vi "UHR-Fleezers Control (host) - 11.0.vi"() -> ()   [LabVIEW 2011] (continued)
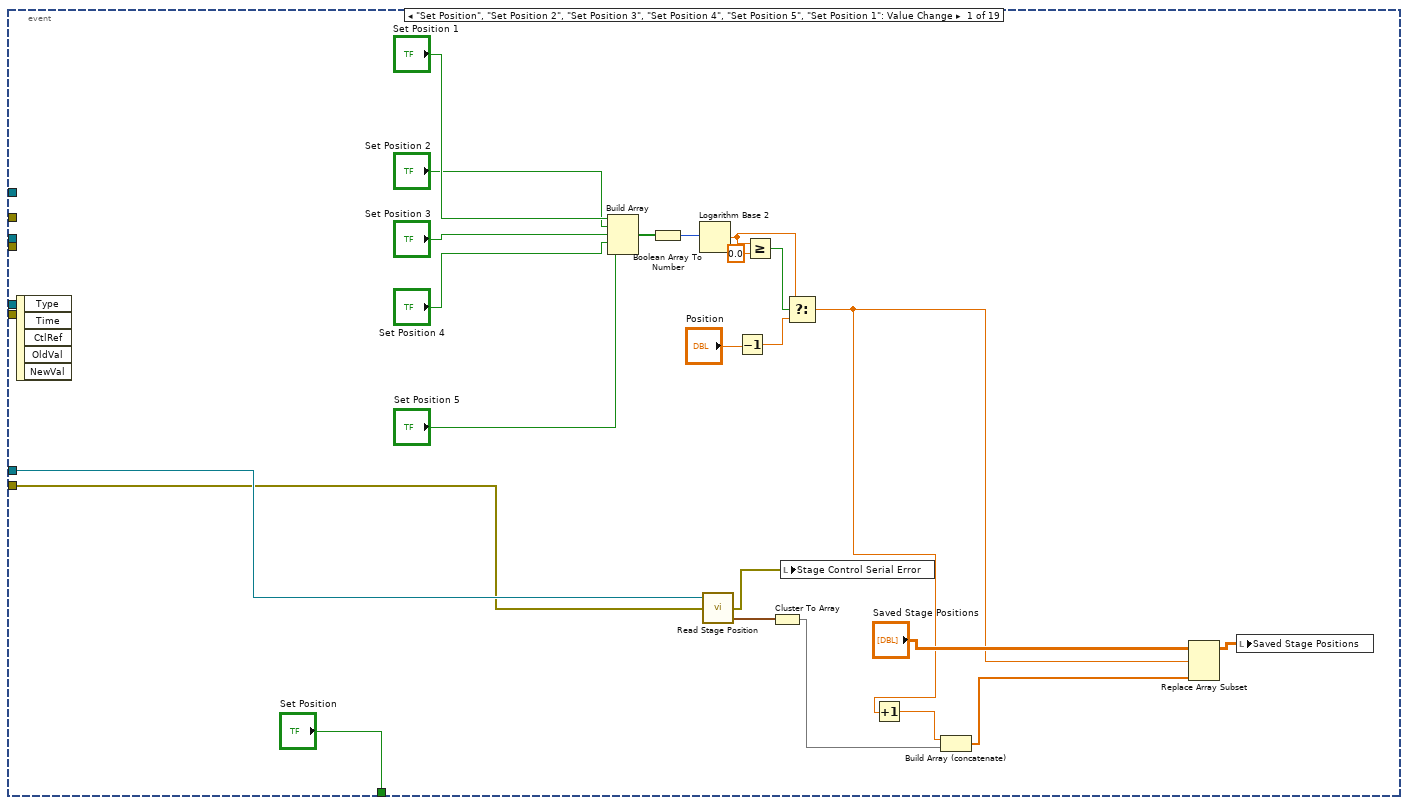
[diagram p2: hidden frame]
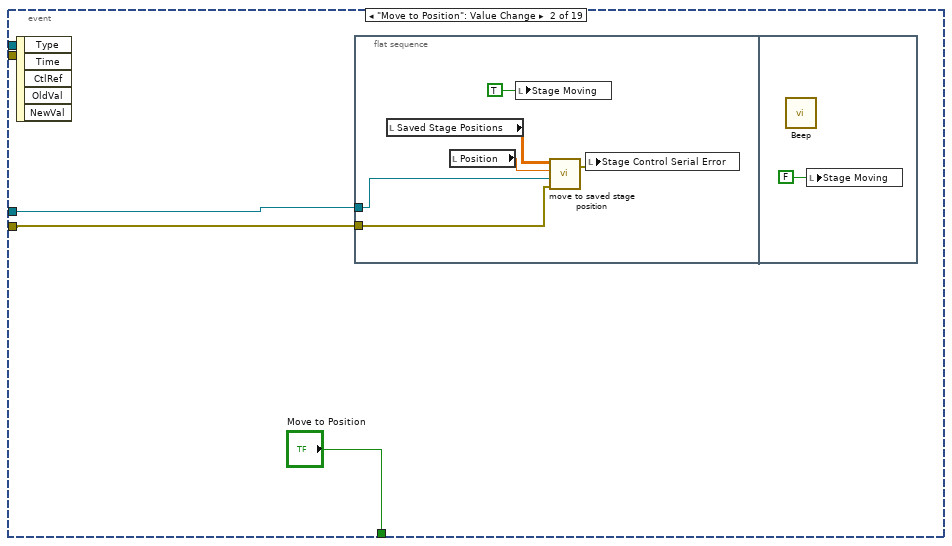
[diagram p3: hidden frame]
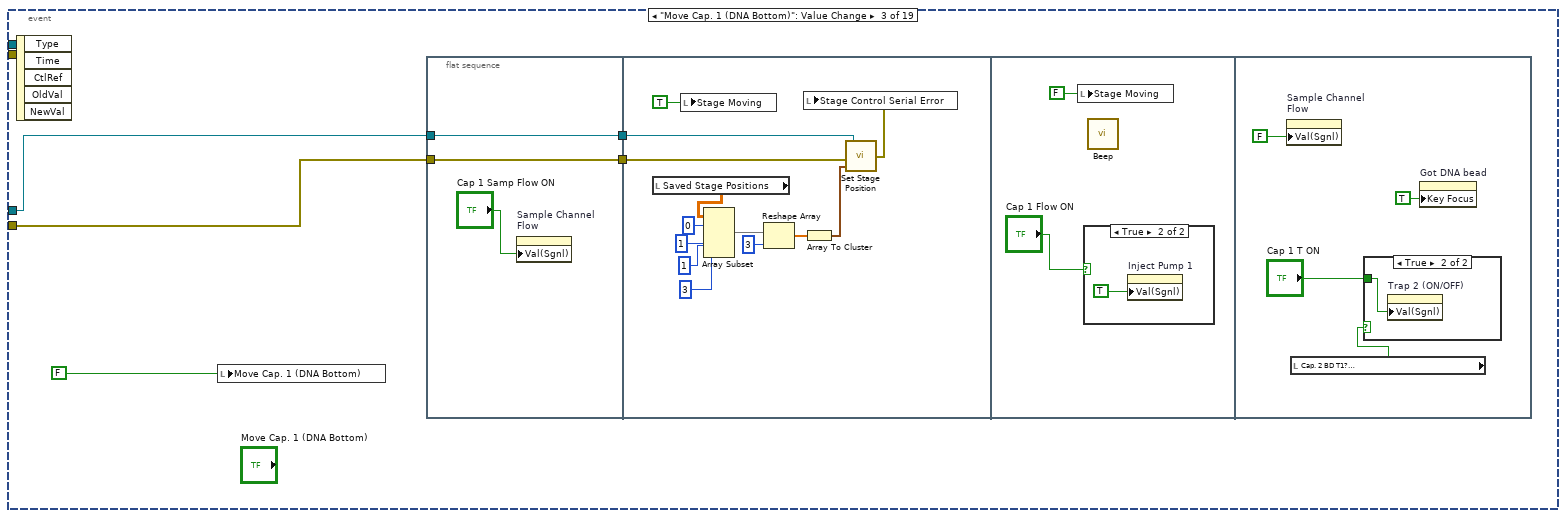
[diagram p4: hidden frame]
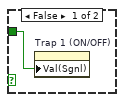
[diagram p6: hidden frame]
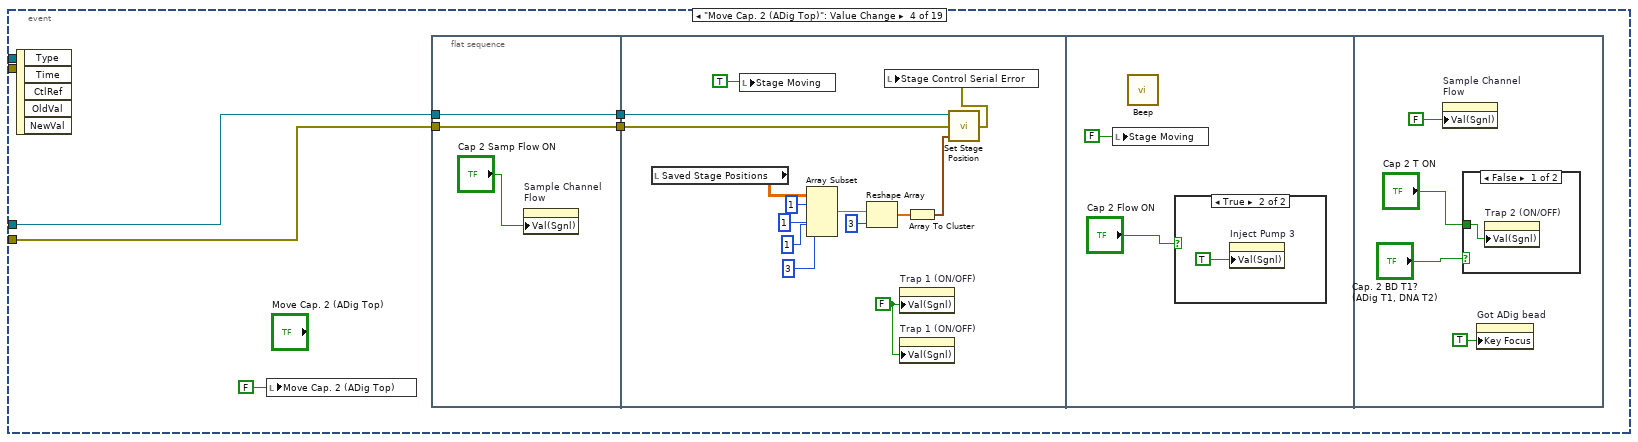
[diagram p7: hidden frame]
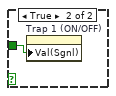
[diagram p9: hidden frame]
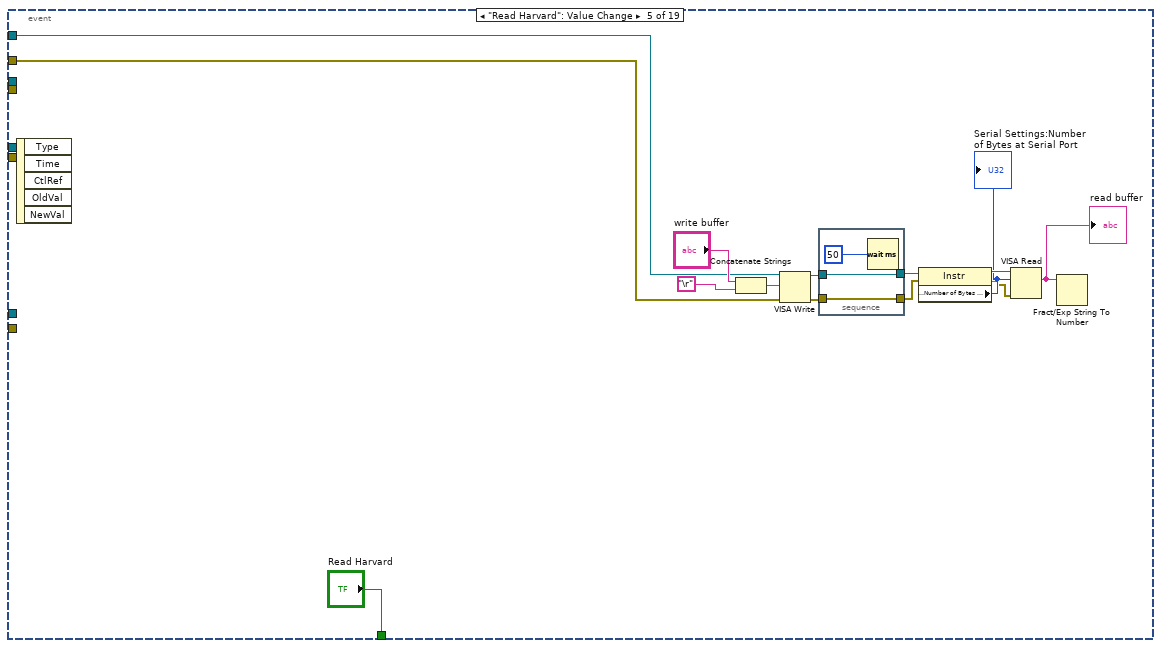
[diagram p10: hidden frame]
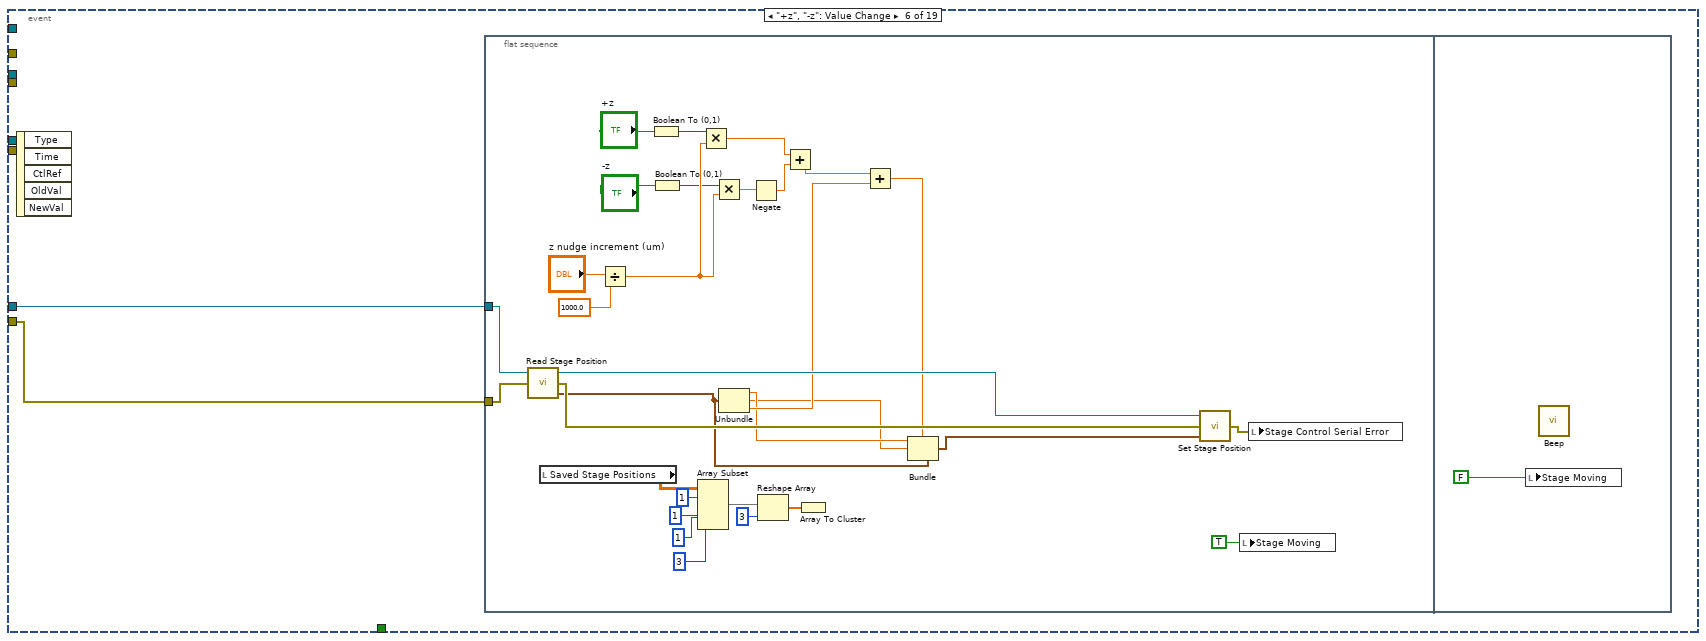
[diagram p11: hidden frame]
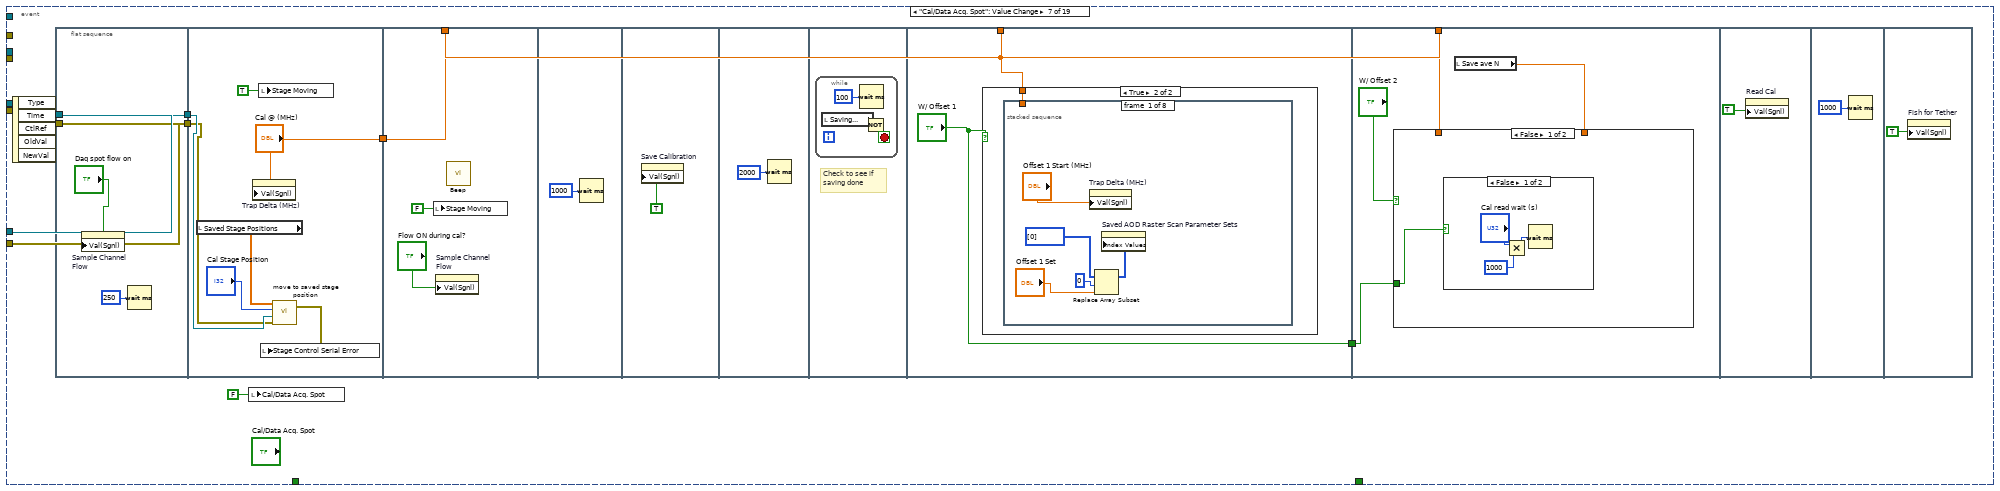
[diagram p12: hidden frame]
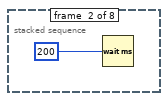
[diagram p14: hidden frame]
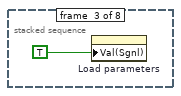
[diagram p15: hidden frame]
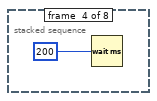
[diagram p16: hidden frame]
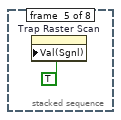
[diagram p17: hidden frame]
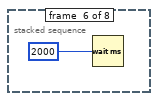
[diagram p18: hidden frame]
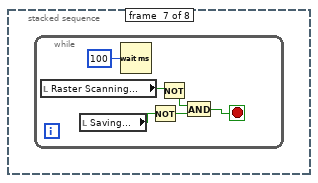
[diagram p19: hidden frame]
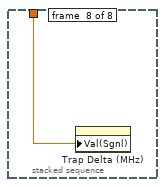
[diagram p20: hidden frame]
                n2907 = Build Array(w4669, w4664, w4662, w4660, w4659, w4650, w4649) -> (w4666:dbl[])
                n2908 = Build Array(w4651, w4655, w4675, w4674, w4673, 3.0 ("t")) -> (w4668:dbl[])
                n2909 = Round Toward +Infinity(x=w4657) -> (ceil(x): smallest int >= x=w4658:dbl)
                n2910 = Build Array (concatenate)(w4668, w4667, w4652, w4666) -> (w4665:dbl[])
                n2911 = To Unsigned Long Integer(number=w4658) -> (unsigned 32bit integer=w4656:u32)
              }
            }
            n2912 = local read "Index"() -> (w4515:dbl)
            n2913 = call "Create new save file.vi"("Insert"="", "Ext"=".dat", "Index In"=w4515) -> ("Path Out"=w4474:path, "Index Out"=w4487:dbl)
            n2914 = local write "Save file name"(w4474) -> ()
            n2915 = local write "Index"(w4487) -> ()
            n2916 = local write "Save index"(w4487) -> ()
            n2917 = Array Size(array=w4498) -> (size(s)=w4499:i32)
            n2918 = Open/Create/Replace File(file path (use dialog)=w4474, operation (0:open)=T25."create", access (0:read/write)=enum16{"read/write", "read-only", "write-only"}."write-only") -> (refnum out=w4512:refnum<file>)  [unwired: 1 in, 4 out]
            n2919 = local write "Saving..."(TRUE ("Saving...")) -> ()
            n2920 = To Double Precision Float(number=w4499) -> (double precision float=w4497:dbl)
            n2921 = String Length(string="Comment (data description)") -> (length=w4495:i32)
            n2922 = To Double Precision Float(number=w4495) -> (double precision float=w4494:dbl)
            n2923 = Deny Access(7:w4512) -> (3:w4511:refnum<file>)  [unwired: 1 in, 2 out]
            n2924 = Build Array (concatenate)(w4497, w4498, w4494) -> (w4496:dbl[])
            n2925 = case "If fluorescence data to be saved" shown="True" w4485 {
              tunnel: w4474 -> [_ w4564]
              tunnel: [refnum<k0> refnum w4544] -> w4486
              frame False {
              }
              frame True {
                w4543 = 0.0
                n2926 = local read "APD Integration Time (s)"() -> (w4549:dbl)
                n2927 = local read "N APD Samp/step"() -> (w4542:dbl)
                n2928 = Path To String(path=w4564) -> (string=w4563:string)
                n2929 = String Length(string=w4563) -> (length=w4562:i32)
                n2930 = Subtract(x=w4562, y=4) -> (x-y=w4560:i32)
                n2931 = String Subset(string=w4563, length (rest)=w4560) -> (substring=w4559:string)  [unwired: 1 out]
                n2932 = Build Array(w4549, w4542, w4543, w4543, w4543, w4543, w4543, w4543) -> (w4546:dbl[])
                n2933 = Concatenate Strings(w4559, "_fl.dat" ("string")) -> (w4557:string)
                n2934 = Array Size(array=w4546) -> (size(s)=w4548:i32)
                n2935 = String To Path(string=w4557) -> (path=w4553:path)
                n2936 = Open/Create/Replace File(file path (use dialog)=w4553, operation (0:open)=T25."create", access (0:read/write)=enum16{"read/write", "read-only", "write-only"}."write-only") -> (refnum out=w4554:refnum<file>)  [unwired: 1 in, 4 out]
                n2937 = Deny Access(7:w4554) -> (3:w4550:refnum<file>)  [unwired: 1 in, 2 out]
                n2938 = To Double Precision Float(number=w4548) -> (double precision float=w4547:dbl)
                n2939 = Build Array (concatenate)(w4547, w4546) -> (w4545:dbl[])
                n2940 = Write to Binary File(file (use dialog)=w4550, data=w4545, 5:FALSE ("prepend array or string size? (T)"), 9:T24."big-endian, network order" ("byte order (0:big-endian, network order)")) -> (refnum out=w4544:refnum<file>)  [unwired: 1 in, 3 out]
              }
            }
            n2941 = case shown="True" w4472 {
              tunnel: w4474 -> [_ w4526]
              tunnel: [refnum<k0> refnum w4525] -> w4473
              frame False {
              }
              frame True {
                w4521 = 0.0 ("element")
                n2942 = Path To String(path=w4526) -> (string=w4540:string)
                n2943 = Build Array(w4521, w4521, w4521, w4521, w4521, w4521, w4521, w4521) -> (w4522:dbl[])
                n2944 = String Length(string=w4540) -> (length=w4539:i32)
                n2945 = Subtract(x=w4539, y=4) -> (x-y=w4537:i32)
                n2946 = Array Size(array=w4522) -> (size(s)=w4524:i32)
                n2947 = String Subset(string=w4540, length (rest)=w4537) -> (substring=w4536:string)  [unwired: 1 out]
                n2948 = To Double Precision Float(number=w4524) -> (double precision float=w4523:dbl)
                n2949 = Concatenate Strings(w4536, "_pos.dat" ("string")) -> (w4534:string)
                n2950 = Build Array (concatenate)(w4523, w4522) -> (w4520:dbl[])
                n2951 = String To Path(string=w4534) -> (path=w4530:path)
                n2952 = Open/Create/Replace File(file path (use dialog)=w4530, operation (0:open)=T25."create", access (0:read/write)=enum16{"read/write", "read-only", "write-only"}."write-only") -> (refnum out=w4531:refnum<file>)  [unwired: 1 in, 4 out]
                n2953 = Deny Access(7:w4531) -> (3:w4527:refnum<file>)  [unwired: 1 in, 2 out]
                n2954 = Write to Binary File(file (use dialog)=w4527, data=w4520, 5:FALSE ("prepend array or string size? (T)"), 9:T24."big-endian, network order" ("byte order (0:big-endian, network order)")) -> (refnum out=w4525:refnum<file>)  [unwired: 1 in, 3 out]
              }
            }
            n2955 = Write to Binary File(file (use dialog)=w4511, data=w4496, 5:w4492, 9:w4490) -> (refnum out=w4493:refnum<file>)  [unwired: 1 in, 3 out]
            n2956 = Write to Binary File(file (use dialog)=w4493, data="Comment (data description)", 5:w4492, 9:w4490) -> (refnum out=w4489:refnum<file>)  [unwired: 1 in, 3 out]
          }
        }
        n2957 = feedback-in #28(w4432) -> ()
        n2958 = feedback-in #29(w4459) -> ()
        n2959 = feedback-in #30(w4431) -> ()
        n2960 = feedback-in #31(w4442) -> ()
        n2961 = feedback-in #32(w4445) -> ()
        n2962 = feedback-in #33(w4458) -> ()
        n2963 = feedback-in #34(w4448) -> ()
      }
      frame #1 {
        n2964 = local read "Saving..."() -> (w4689:bool)
        n2965 = case shown="True" w4689 {
          tunnel: w4693 -> [_ w4703]
          tunnel: w4692 -> [_ w4717]
          tunnel: w4691 -> [_ w4713]
          tunnel: w4690 -> [_ w4712]
          tunnel: w4688 -> [_ w4711]
          tunnel: w4687 -> [_ w4706]
          tunnel: w4686 -> [_ w4705]
          tunnel: w4685 -> [_ w4704]
          tunnel: w4684 -> [_ w4702]
          tunnel: w4683 -> [_ w4700]
          tunnel: w4682 -> [_ w4699]
          tunnel: w4681 -> [_ w4698]
          tunnel: w4680 -> [_ w4697]
          tunnel: w4679 -> [_ w4696]
          tunnel: w4678 -> [_ w4695]
          tunnel: w4677 -> [_ w4694]
          frame False {
          }
          frame True {
            n2966 = Multiply(x=w4703, y=w4702) -> (x*y=→"Time (s)":dbl)
            n2967 = Less Or Equal?(x=w4703, y=w4711) -> (x <= y?=w4715:bool)
            n2968 = Or(x="Stop Saving", y="Abort save 2") -> (x .or. y?=w4707:bool)
            n2969 = Not(x=w4707) -> (.not. x?=w4716:bool)
            n2970 = And(x=w4715, y=w4716) -> (x .and. y?=w4714:bool)
            n2971 = case shown="True" w4714 {
              tunnel: w4717 -> [w4724 w4792]
              tunnel: [0.0 w4795] -> w4710
              tunnel: w4703 -> [_ w4793]
              tunnel: w4711 -> [_ w4794]
              tunnel: w4713 -> [_ w4789]
              tunnel: w4712 -> [_ _]
              tunnel: w4706 -> [w4722 w4782]
              tunnel: w4705 -> [w4721 w4783]
              tunnel: w4704 -> [_ w4781]
              tunnel: w4700 -> [_ w4780]
              tunnel: w4699 -> [_ w4734]
              tunnel: w4698 -> [_ w4773]
              tunnel: w4697 -> [_ w4751]
              tunnel: w4696 -> [w4718 w4732]
              tunnel: w4695 -> [w4719 w4731]
              tunnel: w4694 -> [_ w4728]
              frame False {
                w4720 = FALSE
                n2972 = Close File(refnum=w4724) -> ()  [unwired: 1 in, 2 out]
                n2973 = case shown="True" w4721 {
                  tunnel: w4722 -> [_ w4726]
                  frame False {
                  }
                  frame True {
                    n2974 = Close File(refnum=w4726) -> ()  [unwired: 1 in, 2 out]
                  }
                }
                n2975 = case shown="True" w4718 {
                  tunnel: w4719 -> [_ w4725]
                  frame False {
                  }
                  frame True {
                    n2976 = Close File(refnum=w4725) -> ()  [unwired: 1 in, 2 out]
                  }
                }
                n2977 = local write "Raster Scanning..."(w4720) -> ()
                n2978 = local write "Calibrating Trap..."(w4720) -> ()
                n2979 = call <vilib>:"Beep.vi"() -> ()  [unwired: 3 in, 9 out]
                n2980 = local write "Stop Saving"(w4720) -> ()
                "Saving..." <- w4720
              }
              frame True {
                n2981 = local read "Calibrating Trap..."() -> (w4784:bool)
                n2982 = case "Write fl. data" shown="True" w4783 {
                  tunnel: w4782 -> [_ w4818]
                  tunnel: w4781 -> [_ w4817]
                  frame False {
                  }
                  frame True {
                    n2983 = Write to Binary File(file (use dialog)=w4818, data=w4817, 5:FALSE ("prepend array or string size? (T)"), 9:T24."big-endian, network order" ("byte order (0:big-endian, network order)")) -> ()  [unwired: 1 in, 4 out]
                  }
                }
                n2984 = Greater?(x="Save ave N", y=1.0) -> (0:w4787:bool)
                n2985 = Not(x=w4784) -> (.not. x?=w4786:bool)
                n2986 = And(x=w4786, y=w4787) -> (x .and. y?=w4729:bool)
                n2987 = case shown="True" w4729 {
                  tunnel: w4728 -> [w4798 w4809]
                  tunnel: [w4798 w4801] -> w4727
                  tunnel: "Save ave N" -> [_ w4802]
                  frame False {
                  }
                  frame True {
                    w4799 = 2 ("dimension size")
                    n2988 = Array Size(array=w4809) -> (size(s)=w4803:i32)
                    n2989 = Divide(x=w4803, y=w4799) -> (x/y=w4807:dbl)
                    n2990 = Reshape Array(w4809, w4807, w4799) -> (w4808:u64[][])
                    n2991 = Transpose 2D Array(2D array=w4808) -> (transposed array=w4806:u64[][])
                    n2992 = for {
                      tunnel: w4806 -> [w4811] mode=indexing
                      tunnel: [w4810] -> w4800 mode=indexing
                      tunnel: w4802 -> [w4812]
                      workers-P: _ -> [_]
                      n2993 = call "downsample 1D array - U64.vi"("Ave N"=w4812, "Array In"=w4811) -> ("Array Out"=w4810:u64[])  [unwired: 1 in]
                    }
                    n2994 = Transpose 2D Array(2D array=w4800) -> (transposed array=w4805:u64[][])
                    n2995 = Divide(x=w4803, y=w4802) -> (x/y=w4804:dbl)
                    n2996 = Reshape Array(w4805, w4804) -> (w4801:u64[])
                  }
                }
                n2997 = case shown="False" w4729 {
                  tunnel: w4789 -> [w4821 w4833]
                  tunnel: [w4821 w4825] -> w4785
                  tunnel: "Save ave N" -> [_ w4826]
                  tunnel: w4780 -> [_ w4824]
                  frame False {
                  }
                  frame True {
                    n2998 = Array Size(array=w4833) -> (size(s)=w4827:i32)
                    n2999 = Array Size(array=w4824) -> (size(s)=w4823:i32)
                    n3000 = Divide(x=w4827, y=w4823) -> (x/y=w4831:dbl)
                    n3001 = Reshape Array(w4833, w4831, w4823) -> (w4832:i16[][])
                    n3002 = Transpose 2D Array(2D array=w4832) -> (transposed array=w4830:i16[][])
                    n3003 = for {
                      tunnel: w4830 -> [w4836] mode=indexing
                      tunnel: [w4835] -> w4822 mode=indexing
                      tunnel: w4826 -> [w4834]
                      workers-P: _ -> [_]
                      n3004 = call "downsample 1D array - I16.vi"("Ave N"=w4834, "Array In"=w4836) -> ("Array Out"=w4835:i16[])  [unwired: 1 out]
                    }
                    n3005 = Transpose 2D Array(2D array=w4822) -> (transposed array=w4829:i16[][])
                    n3006 = Divide(x=w4827, y=w4826) -> (x/y=w4828:dbl)
                    n3007 = Reshape Array(w4829, w4828) -> (w4825:i16[])
                  }
                }
                n3008 = Index Array(array=w4751, index=1) -> (element=w4754:waveform(dbl))
                n3009 = Index Array(array=w4751, index=0) -> (element=w4756:waveform(dbl))
                n3010 = Unbundle By Name(w4754) -> ("Y"=w4758:dbl[])
                n3011 = Unbundle By Name(w4756) -> ("Y"=w4766:dbl[])
                n3012 = case "Write trap pos. data" shown="True" w4732 {
                  tunnel: w4731 -> [_ w4814]
                  tunnel: w4727 -> [_ w4813]
                  frame False {
                  }
                  frame True {
                    n3013 = Write to Binary File(file (use dialog)=w4814, data=w4813, 5:FALSE ("prepend array or string size? (T)"), 9:T24."big-endian, network order" ("byte order (0:big-endian, network order)")) -> ()  [unwired: 1 in, 4 out]
                  }
                }
                n3014 = Write to Binary File(file (use dialog)=w4792, data=w4785, 5:FALSE ("prepend array or string size? (T)"), 9:T24."big-endian, network order" ("byte order (0:big-endian, network order)")) -> ()  [unwired: 1 in, 4 out]
                n3015 = feedback #35(w4758) -> (w4760:dbl[])
                n3016 = Build Array (concatenate)(w4760, w4758) -> (w4759:dbl[])
                n3017 = Select(t=w4758, s=w4734, f=w4759) -> (s? t:f=w4744:dbl[])
                n3018 = feedback-in #35(w4744) -> ()
                n3019 = feedback #36(w4766) -> (w4779:dbl[])
                n3020 = Build Array (concatenate)(w4779, w4766) -> (w4778:dbl[])
                n3021 = Select(t=w4766, s=w4734, f=w4778) -> (s? t:f=w4753:dbl[])
                n3022 = feedback-in #36(w4753) -> ()
                n3023 = Divide(x=w4793, y=w4794) -> (x/y=w4796:dbl)
                n3024 = Multiply(x=w4796, y=100.0) -> (x*y=w4795:dbl)
                n3025 = Build Array(w4753, w4744) -> (→"Saved APD":dbl[][])
                n3026 = Array Size(array=w4753) -> (size(s)=w4771:i32)
                n3027 = Unbundle By Name(w4773) -> ("Y"=w4777:dbl[])
                n3028 = Subtract(x=w4771, y="N pts to average") -> (x-y=w4747:i32)
                n3029 = Multiply(x="N pts to average", y=u16 2) -> (x*y=w4748:u16)
                n3030 = Subtract(x=w4771, y=w4748) -> (x-y=w4746:i32)
                n3031 = feedback #37(w4777) -> (w4776:dbl[])
                n3032 = Build Array (concatenate)(w4776, w4777) -> (w4775:dbl[])
                n3033 = Select(t=w4777, s=w4734, f=w4775) -> (s? t:f=w4774:dbl[])
                "Trap Delta Graph" <- w4774
                n3034 = feedback-in #37(w4774) -> ()
                n3035 = Array Subset(array=w4753, index=w4747, length="N pts to average") -> (w4770:dbl[])
                n3036 = Array Subset(array=w4753, index=w4746, length="N pts to average") -> (w4769:dbl[])
                n3037 = Array Subset(array=w4744, index=w4747, length="N pts to average") -> (w4750:dbl[])
                n3038 = Array Subset(array=w4744, index=w4746, length="N pts to average") -> (w4749:dbl[])
                n3039 = call <vilib>:"Mean.vi"("X"=w4770) -> ("mean"=w4768:dbl)  [unwired: 1 out]
                n3040 = call <vilib>:"Mean.vi"("X"=w4750) -> ("mean"=w4743:dbl)  [unwired: 1 out]
                n3041 = call <vilib>:"Mean.vi"("X"=w4769) -> ("mean"=w4767:dbl)  [unwired: 1 out]
                n3042 = call <vilib>:"Mean.vi"("X"=w4749) -> ("mean"=w4742:dbl)  [unwired: 1 out]
                n3043 = Subtract(x=w4743, y=w4742) -> (x-y=w4733:dbl)
                "Delta Fl. 2" <- w4733
                n3044 = Subtract(x=w4768, y=w4767) -> (x-y=w4765:dbl)
                "Delta Fl. 1" <- w4765
                n3045 = Initialize Array(w4765, 1 ("dimension size")) -> (w4762:dbl[])
                n3046 = Initialize Array(w4733, 1 ("dimension size")) -> (w4739:dbl[])
                n3047 = feedback #38(w4762) -> (w4763:dbl[])
                n3048 = Build Array (concatenate)(w4763, w4762) -> (w4761:dbl[])
                n3049 = feedback #39(w4739) -> (w4740:dbl[])
                n3050 = Build Array (concatenate)(w4740, w4739) -> (w4738:dbl[])
                n3051 = Select(t=w4762, s=w4734, f=w4761) -> (s? t:f=w4737:dbl[])
                n3052 = feedback-in #38(w4737) -> ()
                n3053 = Select(t=w4739, s=w4734, f=w4738) -> (s? t:f=w4736:dbl[])
                n3054 = feedback-in #39(w4736) -> ()
                n3055 = Build Array(w4737, w4736) -> (→"Save APD Deriv":dbl[][])
              }
            }
            "Progress" <- w4710
            "Progress 2" <- w4710
          }
        }
      }
    }
    n3056 = Bundle By Name(cluster=w3372, "Green FB Ch 0"=w3371, "Green FB Ch 1"=w3370) -> (w3350:T47)
    "Green FB Signals (V)" <- w3350
    n3057 = Unbundle By Name(w3350) -> ("Green FB Ch 2"=→"Green FB Plot":dbl)
    n3058 = local read "wait to reset values"() -> (w3441:bool)
    n3059 = Not(x=w3439) -> (.not. x?=w3442:bool)
    n3060 = And(x=w3442, y=w3441) -> (x .and. y?=w3443:bool)
    n3061 = case "Part of MCL raster scanning: returns to initial positions after scan done" shown="True" w3443 {
      tunnel: w3156 -> [w4252 w4259]
      tunnel: [w4252 w4258] -> w3445
      tunnel: w3155 -> [w4251 w4257]
      tunnel: [w4251 w4256] -> w3440
      frame False {
      }
      frame True {
        w4267 = 10.0 ("y")
        w4266 = 32767.0 ("y")
        # "to return scan values\nafter a synchronous \nAOM scan"
        n3062 = local read "AO2"() -> (w4260:dbl)
        n3063 = local read "AO1"() -> (w4261:dbl)
        n3064 = local write "wait to reset values"(FALSE ("wait to reset values")) -> ()
        n3065 = Multiply(x=w4261, y=w4266) -> (x*y=w4263:dbl)
        n3066 = Multiply(x=w4260, y=w4266) -> (x*y=w4265:dbl)
        n3067 = Divide(x=w4263, y=w4267) -> (x/y=w4262:dbl)
        n3068 = Divide(x=w4265, y=w4267) -> (x/y=w4264:dbl)
        n3069 = To Word Integer(number=w4262) -> (16bit integer=w4268:i16)
        n3070 = To Word Integer(number=w4264) -> (16bit integer=w4269:i16)
        n3071 = local read "Total Counts (ticks)"() -> (w4253:u32)
        n3072 = xnode "Read/Write Control"("FPGA VI Reference In"=w4259, "error in"=w4257, "AO1"=w4268, "AO2"=w4269, "MCL count"=w4253) -> ("FPGA VI Reference Out"=w4258:T19, "error out"=w4256:errorcluster)
        n3073 = local read "Scan Range (V)\n(of steps)"() -> (w4254:dbl)
        n3074 = property on="Scan Range (V)\n(of steps)" class="DigNum (strict)"("Val(Sgnl)"=w4254) -> ()  [unwired: 2 in, 2 out]
      }
    }
    n3075 = node-c288() -> ()  [unwired: 2 out]
  }
  n3076 = VISA Close(VISA resource name=w82, error in (no error)=w81) -> (error out=w130:errorcluster)
  n3077 = call <vilib>:"Simple Error Handler.vi"("error in (no error)"=w130) -> ()  [unwired: 1 in, 8 out]
  n3078 = node-c288(w89) -> ()  [unwired: 1 out]
  n3079 = node-c288(w174) -> ()  [unwired: 1 out]
  n3080 = flat-sequence {
    tunnel: w268 -> [w4840]
    tunnel: w270 -> [w4841]
    tunnel: [w4839] -> w249
    tunnel: [w4838] -> w248
    tunnel: w230 -> [_]
    tunnel: w182 -> [_]
    tunnel: w95 -> [_]
    tunnel: w249 -> [w4842]
    tunnel: w248 -> [w4843]
    frame #0 {
      w4837 = FALSE ("AI to FIFO")
      n3081 = xnode "Read/Write Control"("FPGA VI Reference In"=w4841, "error in"=w4840, "AI to FIFO"=w4837, "APD to FIFO"=w4837) -> ("FPGA VI Reference Out"=w4839:T19, "error out"=w4838:errorcluster)
    }
    frame #1 {
      n3082 = xnode "Close FPGA VI Reference"("FPGA VI Reference In"=w4842, "error in"=w4843) -> ("error out"=→"error out":errorcluster)
    }
  }
